vi "Untitled 1.vi"() -> ()   [LabVIEW 2020]
uses:
  <vilib>/Instr/_visa.llb/VISA Configure Serial Port (Instr).vi
panel:
  in  "String":string
  in  "stop":bool
  in  "Boolean":bool
  in  "VISA resource name":refnum<visa-resource-name>
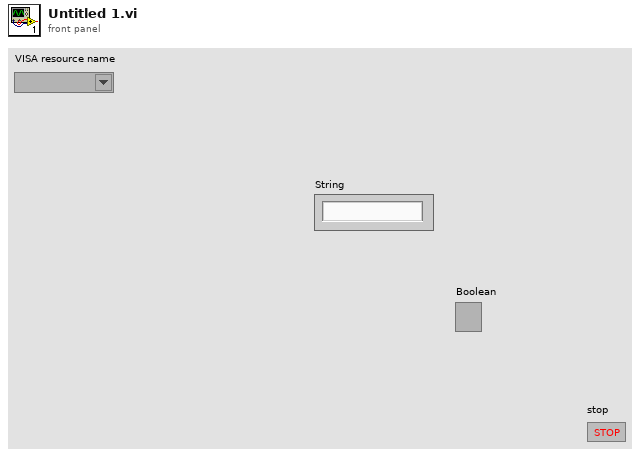
[diagram p1: front panel]
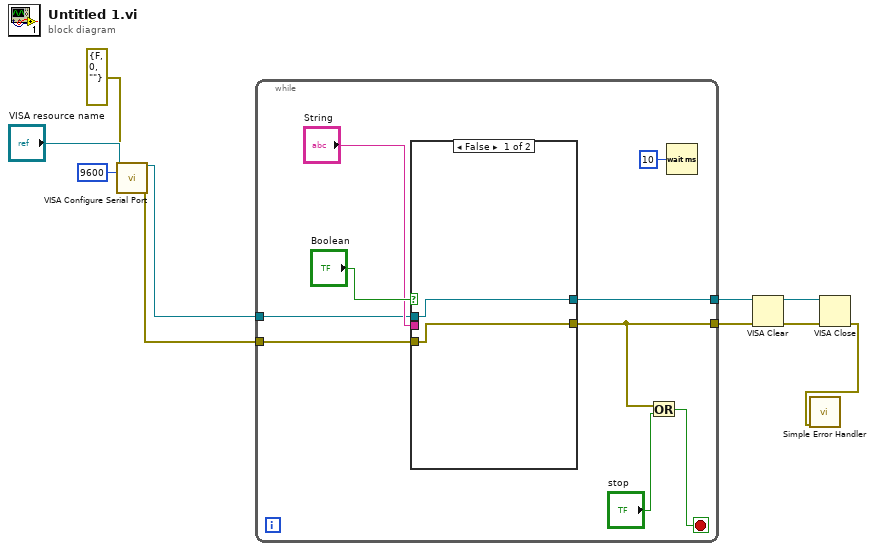
[diagram p0: block diagram]
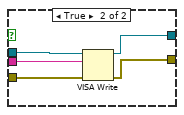
[diagram p2: hidden frame]
diagram:
  n1 = call-poly "VISA Configure Serial Port"("VISA resource name"="VISA resource name", "baud rate (9600)"=u32 9600, "error in (no error)"=errorcluster {"status"=FALSE, "code"=0, "source"=""}) -> ("VISA resource name out"=w8:refnum<visa-resource-name>, "error out"=w7:errorcluster)  [unwired: 11 in]
  n2 = while {
    tunnel: [w17] -> w4
    tunnel: [w13] -> w2
    tunnel: w8 -> [w16]
    tunnel: w7 -> [w15]
    stop <- w11 stop-if-true
    n3 = case shown="False" "Boolean" {
      tunnel: "String" -> [_ w26]
      tunnel: [w21 w25] -> w17
      tunnel: [w20 w24] -> w13
      tunnel: w16 -> [w21 w23]
      tunnel: w15 -> [w20 w22]
      frame False {
      }
      frame True {
        n4 = VISA Write(VISA resource name=w23, write buffer=w26, error in (no error)=w22) -> (VISA resource name out=w25:refnum<visa-resource-name>, error out=w24:errorcluster)  [unwired: 1 out]
      }
    }
    n5 = Or(x=w13, y="stop") -> (x .or. y?=w11:bool)
    n6 = Wait (ms)(milliseconds to wait=u32 10) -> ()  [unwired: 1 out]
  }
  n7 = VISA Clear(VISA resource name=w4, error in (no error)=w2) -> (VISA resource name out=w3:refnum<visa-resource-name>, error out=w1:errorcluster)
  n8 = VISA Close(VISA resource name=w3, error in (no error)=w1) -> (error out=w5:errorcluster)
  n9 = call <vilib>:"Simple Error Handler.vi"("error in (no error)"=w5) -> ()  [unwired: 4 in, 5 out]
